vi "Activate.vi"(5 "DO Task":refnum<k21>, 7 "AO Task":refnum<k21>, 8 "error constant":errorcluster, 10 "AO":T1(array[cluster]), 11 "DO":T2(array[cluster])=[{"CDT"=-150.0, "Position"=TRUE, "Component ID"="F_EPV_131"}, {"CDT"=-150.0, "Position"=TRUE, "Component ID"="F_EPV_131"}, {"CDT"=-135.0, "Position"=FALSE, "Component ID"="F_EPV_132"}, {"CDT"=-120.0, "Position"=FALSE, "Component ID"="F_EPV_131"}, {"CDT"=-20.0, "Position"=TRUE, "Component ID"="F_EPV_136"}, {"CDT"=-10.0, "Position"=FALSE, "Component ID"="F_EPV_136"}]) -> (0 "error out":errorcluster, 3 "Abort":bool)   [LabVIEW 2022 SP3]
uses:
  <vilib>/Platform/TimedLoop/XDataNode/timing_clust.ctl
  <vilib>/Platform/TimedLoop/XDataNode/nitl_modes.ctl
  <vilib>/Platform/TimedLoop/XDataNode/wakeup.ctl
  RT Controls/DO FGV.ctl
  RT Controls/AO FGV.ctl
  <vilib>/DAQmx/write.llb/DAQmx Write (Digital 1D Bool NChan 1Samp 1Line).vi
  <vilib>/DAQmx/write.llb/DAQmx Write (Analog 1D DBL 1Chan NSamp).vi
  RT Sub VI's/RT Global.vi
  <vilib>/DAQmx/miscellaneous.llb/DAQmx Fill In Error Info.vi
  <vilib>/platform/TimedLoop/XDataNode/XDataNode.xnode
  <vilib>/Platform/TimedLoop/XDataNode/XDNodeRunTimeDep.lvlib
panel:
  out "y":dbl
  in  "Launch Time":timestamp
  out "x":u32
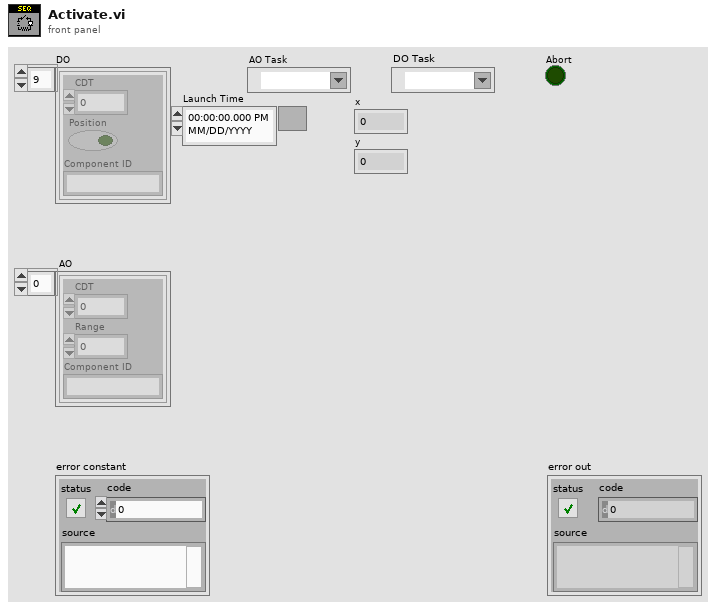
[diagram p1: front panel]
types:
  T1 = cluster{"CDT":dbl, "Range":dbl, "Component ID":string}[]
  T2 = cluster{"CDT":dbl, "Position":bool, "Component ID":string}[]
  T3 = cluster{"AO":cluster{"CDT":dbl, "Range":dbl, "Component ID":string}[], "DO":cluster{"CDT":dbl, "Position":bool, "Component ID":string}[], "Launch Time":timestamp}
  T4 = typedef "XDNodeRunTimeDep.lvlib/timing_clust.ctl" = cluster{"Expected End [f-1]":u64, "Actual End [f-1]":u64, "Finished Late? [f-1]":bool, "Expected End [i-1]":u64, "Actual End [i-1]":u64, "Finished Late? [i-1]":bool, "Expected Start [i]":u64, "Actual Start [i]":u64, "Expected Start [f]":u64, "Actual Start [f]":u64, "Source Name":string, "Structure Name":string, "Period":i64, "Deadline":i64, "Offset":i64, "Start":i64, "Priority":i32, "Timeout":i32, "Mode":T5, "Wakeup Reason":T6, "Error":errorcluster, "Source Type":string, "Secondary Source Type":string, "Global End Time":u64, "Global Start Time":u64, "Frame Duration":u64, "Iteration Duration":u64, "Assigned CPU":i32, "I/O Scan Engine Mode":u32}
  T5 = typedef "XDNodeRunTimeDep.lvlib/nitl_modes.ctl" = enum32{"No Change", "Process missed periods, maintain original phase", "Discard missed periods, maintain original phase", "Process missed periods, ignore original phase", "Discard missed periods, ignore original phase"}
  T6 = typedef "XDNodeRunTimeDep.lvlib/wakeup.ctl" = enum32{"Normal", "Aborted", "Asynchronous wakeup", "Timing source error", "Timed loop error", "Timeout"}
  T7 = typedef "AO FGV.ctl" = enum16{"Read", "Write", "Start time", "init", "Read Only"}
  T8 = typedef "DO FGV.ctl" = enum16{"Read", "Write", "Start time", "init", "Read only"}
  T9 = cluster{"CDT":dbl, "Position":bool, "Component ID":string}
  T10 = cluster{"CDT":dbl, "Range":dbl, "Component ID":string}
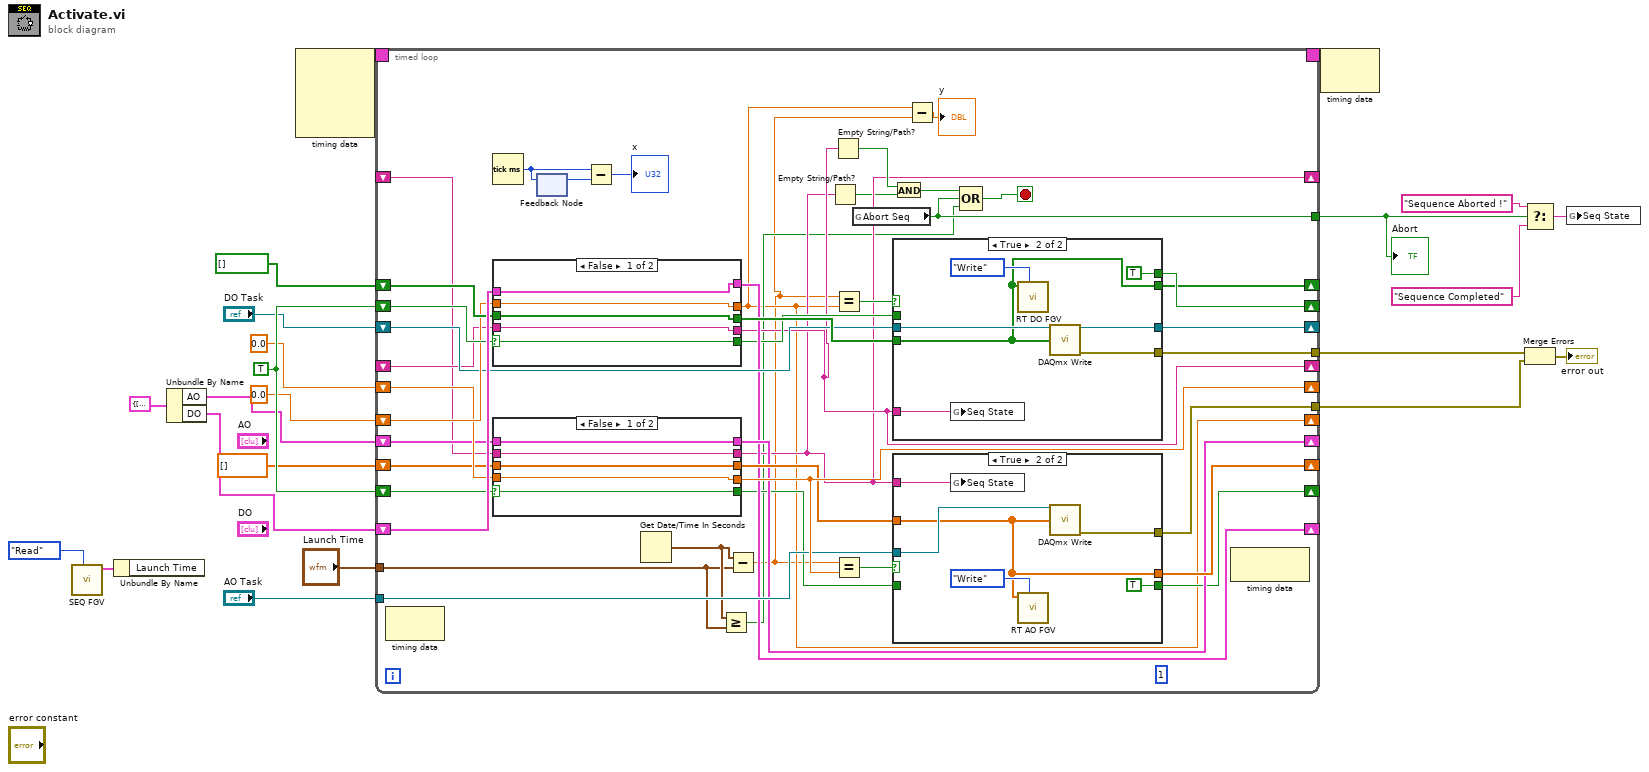
[diagram p0: block diagram]
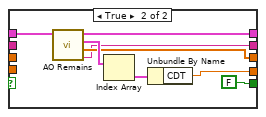
[diagram p3: hidden frame]
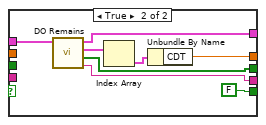
[diagram p5: hidden frame]
diagram:
  w22 = TRUE
  n1 = call "SEQ FGV.vi"("Enum"=enum16{"Read", "Write"}."Read") -> ("Seq data out"=w14:T3)  [unwired: 9 in, 1 out]
  n2 = Unbundle By Name(w14) -> ()  [unwired: 1 out]
  n3 = Unbundle By Name(T3 {"AO"=[{"CDT"=-150.0, "Range"=3.0, "Component ID"="M_PT_1"}, {"CDT"=-120.0, "Range"=3.0, "Component ID"="M_PT_2"}, {"CDT"=-120.0, "Range"=3.0, "Component ID"="M_PT_3"}, {"CDT"=-100.0, "Range"=3.0, "Component ID"="M_PT_4"}, {"CDT"=-50.0, "Range"=3.0, "Component ID"="M_PT_5"}, {"CDT"=-50.0, "Range"=3.0, "Component ID"="M_PT_6"}], "DO"=[{"CDT"=-100.0, "Position"=TRUE, "Component ID"="C_EPV_MOV"}, {"CDT"=-50.0, "Position"=TRUE, "Component ID"="C_EPV_MOV2"}, {"CDT"=-50.0, "Position"=FALSE, "Component ID"="C_EPV_MOV3"}, {"CDT"=-5.0, "Position"=TRUE, "Component ID"="C_EPV_MOV4"}], "Launch Time"=timestamp(3804736718.745 s since 1904-01-01)} ("Seq data out")) -> ("AO"=w3:T1, "DO"=w2:T2)
  n4 = node-c288() -> (w17:T4)  [unwired: 4 in]
  n5 = timed-loop {
    shift-right: [w47] -> _
    shift-left: w2 -> [w66]
    shift-right: [w43] -> _
    shift-left: w22 -> [w65]
    shift-right: [w40] -> _
    shift-left: bool[] [] ("DO value") -> [w64]
    shift-right: [w25] -> _
    shift-left: 0.0 ("CDT") -> [w63]
    shift-right: [w57] -> _
    shift-left: 0.0 ("CDT") -> [w60]
    shift-right: [w48] -> _
    shift-left: w3 -> [w59]
    shift-right: [w41] -> _
    shift-left: w22 -> [w55]
    shift-right: [w50] -> _
    shift-left: dbl[] [] ("AO") -> [w54]
    shift-right: [w52] -> _
    shift-left: "DO Task" -> [w53]
    tunnel: [w38] -> w20
    tunnel: "AO Task" -> [w51]
    tunnel: [w39] -> w6
    timing: w17 -> [_]
    timing-out: [_] -> w16
    tunnel: "Launch Time" -> [w27]
    tunnel: [w37] -> w5
    shift-right: [w31] -> _
    shift-left: _ -> [w36]
    shift-right: [w30] -> _
    shift-left: _ -> [w35]
    stop <- w49 stop-if-true
    (unwired) 1 ("Size")
    n6 = node-c288() -> ()  [unwired: 1 in, 1 out]
    n7 = Tick Count (ms)() -> (millisecond timer value=w33:u32)
    n8 = case shown="False" w65 {
      selector: w65 -> [w101 _]
      tunnel: w66 -> [w102 w112]
      tunnel: [w102 w107] -> w47
      tunnel: [w104 w109] -> w62
      tunnel: w64 -> [w104 _]
      tunnel: [w103 w108] -> w25
      tunnel: w63 -> [w103 _]
      tunnel: [w101 FALSE] -> w44
      tunnel: [w100 w105] -> w31
      tunnel: w36 -> [w100 _]
      frame False {
      }
      frame True {
        n9 = call "DO Remains.vi"("Array"=w112) -> ("Status"=w105:string, "DO value"=w109:bool[], "Same DO"=w111:T2, "Remains"=w107:T2)  [unwired: 7 in]
        n10 = Index Array(array=w111) -> (element=w110:T9)  [unwired: 1 in]
        n11 = Unbundle By Name(w110) -> ("CDT"=w108:dbl)
      }
    }
    n12 = case shown="False" w55 {
      selector: w55 -> [w79 _]
      tunnel: w59 -> [w80 w89]
      tunnel: [w80 w85] -> w48
      tunnel: [w81 w86] -> w57
      tunnel: w60 -> [w81 _]
      tunnel: [w79 FALSE] -> w42
      tunnel: [w78 w83] -> w56
      tunnel: w54 -> [w78 _]
      tunnel: [w77 w82] -> w30
      tunnel: w35 -> [w77 _]
      frame False {
      }
      frame True {
        n13 = call "AO Remains.vi"("Array"=w89) -> ("String"=w82:string, "AO"=w83:dbl[], "Same AO"=w88:T1, "Remains AO"=w85:T1)  [unwired: 7 in]
        n14 = Index Array(array=w88) -> (element=w87:T10)  [unwired: 1 in]
        n15 = Unbundle By Name(w87) -> ("CDT"=w86:dbl)
      }
    }
    n16 = feedback-in #1(w33) -> ()
    n17 = feedback #1() -> (w34:u32)  [unwired: 1 in]
    n18 = Subtract(x=w33, y=w34) -> (x-y=→"x":u32)
    n19 = Get Date/Time In Seconds() -> (seconds since 1Jan1904=w28:timestamp)
    n20 = Greater Or Equal?(x=w28, y=w27) -> (x >= y?=w26:bool)
    n21 = Subtract(x=w28, y=w27) -> (x-y=w24:dbl)
    n22 = Empty String/Path?(string/path=w30) -> (empty?=w29:bool)
    n23 = Empty String/Path?(string/path=w31) -> (empty?=w46:bool)
    n24 = Equal?(x=w24, y=w25) -> (x = y?=w61:bool)
    n25 = Equal?(x=w24, y=w57) -> (x = y?=w58:bool)
    n26 = global read "RT Global.vi" "Abort Seq"() -> (w39:bool)
    n27 = case shown="True" w61 {
      tunnel: w62 -> [w92 w93]
      tunnel: [w92 w93] -> w40
      tunnel: w53 -> [w91 w99]
      tunnel: [w91 w98] -> w52
      tunnel: [_ w97] -> w37
      tunnel: w44 -> [w90 _]
      tunnel: [w90 TRUE] -> w43
      tunnel: w31 -> [_ w95]
      frame False {
      }
      frame True {
        n28 = global write "RT Global.vi" "Seq State"(w95) -> ()
        n29 = call "RT DO FGV.vi"("Enum"=DO_FGV."Write", "DO in"=w93) -> ()  [unwired: 7 in, 3 out]
        n30 = call-poly <vilib>:"DAQmx Write.vi"("task/channels in"=w99, "data"=w93) -> ("task out"=w98:refnum<k21>, "error out"=w97:errorcluster)  [unwired: 11 in, 1 out]
      }
    }
    n31 = case shown="True" w58 {
      tunnel: w56 -> [w70 w71]
      tunnel: [w70 w71] -> w50
      tunnel: [_ w76] -> w38
      tunnel: w51 -> [_ w75]
      tunnel: w42 -> [w69 _]
      tunnel: [w69 TRUE] -> w41
      tunnel: w30 -> [_ w73]
      frame False {
      }
      frame True {
        n32 = global write "RT Global.vi" "Seq State"(w73) -> ()
        n33 = call "RT AO FGV.vi"("Enum"=AO_FGV."Write", "AO in"=w71) -> ()  [unwired: 7 in, 3 out]
        n34 = call-poly <vilib>:"DAQmx Write.vi"("task/channels in"=w75, "data"=w71) -> ("error out"=w76:errorcluster)  [unwired: 11 in, 2 out]
      }
    }
    n35 = And(x=w46, y=w29) -> (x .and. y?=w45:bool)
    n36 = Subtract(x=w25, y=w24) -> (x-y=→"y":dbl)
    n37 = Compound Arithmetic op=OR(w45, w39, w26) -> (w49:bool)
    n38 = node-c288() -> ()  [unwired: 1 in, 1 out]
  }
  "Abort" <- w6
  n39 = node-c288(w16) -> ()  [unwired: 1 out]
  n40 = Select(t="Sequence Aborted !" ("Seq State"), s=w6, f="Sequence Completed" ("Seq State")) -> (s? t:f=w7:string)
  n41 = Merge Errors(w5, w20) -> (→"error out":errorcluster)
  n42 = global write "RT Global.vi" "Seq State"(w7) -> ()
